vi "FestoCPX.Station.Table.Ready.vi"(7 "Log (T)":bool=TRUE, 8 "error in":errorcluster) -> (0 "error out":errorcluster, 2 "Ready state":T1)   [LabVIEW 2016]
uses:
  FestoCPX.Station.Table.ReadyState.ctl
  tools/EventLog/EventLog.EventSource.ctl
  tools/Translator/Translator.Message.ctl
  tools/EventLog/EventLog.CreateError(array).vi
  tools/Translator/Translator.Translate.Status (NoError).vi
  tools/Translator/Translator.FormatMessage.vi
  tools/Translator/Translator.Global.vi
  tools/ErrorHandling/ErrorHandling.Create.vi
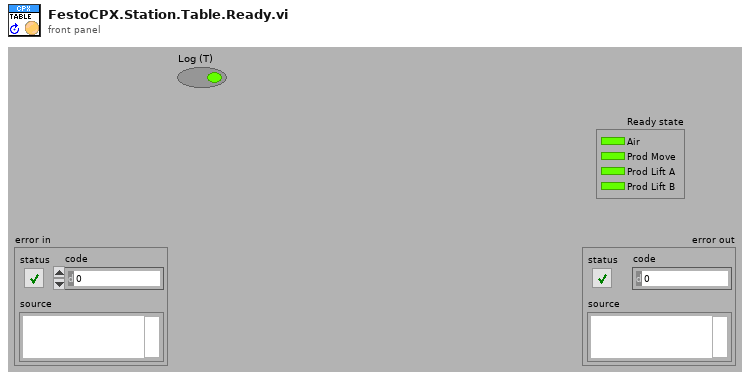
[diagram p1: front panel]
types:
  T1 = typedef "FestoCPX.Station.Table.ReadyState.ctl" = cluster{"Air":bool, "Prod Move":bool, "Prod Lift A":bool, "Prod Lift B":bool}
  T2 = typedef "EventLog.EventSource.ctl" = enum16{"All", "Gui", "Ref", "File", "Arch", "Seq", "CPX", "DB", "Laser", "Scan.P", "Scan.O"}
  T3 = typedef "Translator.Message.ctl" = enum16{"-", "Event confirmed", "Log out", "Log in", "Shutdown", "Cancel", "Start", "Begin time", "End time", "Duration", "Service Mode", "Ignore Results", "Serial Format", "On", "Off", "OK", "NOK", "NOK %s", "Home", "Work", "Close", "Open", "In progress...", "Missing", "Empty", "Hardware failure", "Initial", "Default", "Total", "Out of range", "Free disk space is below 1GB - contact technician", "Error %d >> %s", "Error %d >> %s >> %s", "Msg %d >> %s", "Laser msg %d %s", "Laser cmd error %s %d", "Laser cmd failed %s", "Laser cmd warning %s", "Laser disconnected", "Laser status %s", "Laser already started", "Laser job unkonwn %s", "Laser job missing %s", "Laser job select failure %s", "Unable to start laser printing (%s)", "Unable to stop laser printing (%s)", "Laser marking aborted", "Laser marking timeout", "Unable to reset Laser Interlock (%s)", "Unable to trigger Laser. Laser not ready (%s)", "Laser job '%s' coordinates not configured", "Starting %s", "Quitting %s", "Configured", "Initializing", "Quitting", "Loading", "Loaded %d results", "Loaded %d events", "Running", "Stopped", "Summary", "Laser", "Do you want to continue?", "Do you want to delete the configuration?", "The configuration is being used by an order. Unable to delete!", "Press confirm button", "Station is not based. Do you want to exit?", "Station requires changeover. Do you want to run the test?", "Test options are not set as default. Do you want to continue?", "Formatting of WabcoNo is disabled. Do you want to continue?", "Product not detected. Do you want to continue?", "Product scan failed. Do you want to continue?", "Calibration", "Log out?", "System", "All", "IDLE", "Translating...%s", "Not found", "Alarm %s", "Run", "Skip", "Abort", "Repeat", "Please wait...", "Database disconnected", "Database disconnected - changeover disabled!", "Login to database successful", "Login to database failed: %d; %s", "Unable to check the product status of reference %d - database disconnected", "Unable to set the product status of reference %d - database disconnected", "Variant file backup %s", "Read variant (%s)", "Result", "Station armed!", "Station requires changeover!", "Select reference number...", "EMERGENCY BUTTON - press Control button", "EMERGENCY DOOR - press Control button", "Resetting Emergency...", "Unable to reset safety circuit - Emergency Button pressed", "Unable to reset safety circuit - Emergency Side Door open", "Station not based", "Station based", "Station not empty", "Station basing...", "No order", "Press Start to begin new order", "Scanning new order", "Order NOK. Correct or scan again", "Order OK. Press Accept", "Order ready", "Revolver incorrect", "Fork incorrect", "Revolver missing", "Revolver empty", "Container missing", "Offline results", "Offline statistics", "Updating statistics %.1f %%", "DMC Configurator", "Door open", "Close the front door", "Press start button", "Done. Open the front door", "Running...", "Running...%.1f %%", "Pause %s", "Pause %s. NOK container missing", "Pause %s. OK container missing", "Pause %s. Revolver empty", "Pause %s. Revolver missing", "Pause %s. Revolver incorrect", "Pause %s. Fork missing", "Pause %s. Fork incorrect", "Pause %s. Too many failures", "Pause %s. Unloading failure", "Pause %s. One slot is not working", "Pause %s. Part order is done. Empty OK container", "Pause %s. Unable to move product to slot", "Pause %s. Unable to move back product pusher", "Pause %s. Unable to lift product", "Pause %s. Unable to move back product lifter", "Pause %s. Unable to move product arm to Work", "Pause %s. Unable to move product arm to NOK", "Pause %s. Unable to move product arm to OK", "Pause %s. Unable to unsuck the NOK product", "Pause %s. Unable to drop the NOK product", "Pause %s. Product OK missing", "Pause %s. Unable to unsuck the OK product", "Pause %s. Unable to drop the OK product", "Stopping...", "File '%s' is missing", "File '%s' is broken", "File '%s' is running", "Log file started (%s)", "Log file ended (%s)", "Log file stopped (%s)", "Log file ignored (%s)", "Log file exported (%s)", "Log file export failed (%s)", "Wrong serial number in log file", "Wrong reference number in log file", "Test steps are missing", "%s = %.3f", "Process param '%s' not found in DB", "Process param '%s' wrong order", "Process param '%s' value %.3f out of limits (%.3f; %.3f)", "Step%d param '%s' not found in DB", "Step%d param '%s' wrong order", "Step%d param '%s' value %.3f out of limits (%.3f; %.3f)", "Step%d EV '%s' not found in DB", "Step%d EV '%s' wrong order", "\"%s\" not found in DB", "\"%s\" wrong order", "\"%s\" value %.3f out of limits (%.3f; %.3f)", "\"%s\" not found in software", "Process init (%s)", "Process started", "Process restarted", "Process run", "Process done", "Process done - remove OK container", "Process aborted", "Process aborted at work", "Process aborted at home", "Process error", "Process error at home", "Process error at work", "Process close", "Process pause", "Process continue", "Process door open", "Process door close", "Process pause at slot %s due to %s", "Select plate from the order to process", "Do you want to start the process?", "Do you want to continue the process?", "There is unfinished order. Do you want to put the new order?", "Product %s %d OK", "Product %s %d NOK", "Unable to unload the slot %s. Product missing in the slot", "Unable to unload the slot %s. Product already in the arm", "Unable to accept the product as OK. Product missing in slot %s", "Unable to accept the product as OK. Product could not drop into the container at slot %s", "Unable to accept the product as NOK. Product could not drop into the container at slot %s", "Scan failed. Error %s", "Scan failed. Scanner disconnected", "Scan failed. Wrong Wabco number %d, limit (%d,%d)", "Scan failed. Wrong serial number %d, limit (%d,%d)", "Scan failed. Wrong date %d, limit (%d,%d)", "Scan failed. Wrong product wabco number %d (expected %d)", "Scan failed. Wrong product serial number %d (expected > 0)", "Scan OK %s", "Scan failed. Unable to determine table position (%s)", "Scan failed. Timeout", "Tune failed. Scanner disconnected", "Tune failed. Timeout", "%s = %d", "%s = %d->%d", "Unable to set %s = %.2f - Air Pressure Inside off", "Unable to set digital output '%s' = %d", "Unable to activate air pressure inside - timeout", "Unable to activate air pressure inside - aborted", "Unable to switch on Air Main Valve - Air Pressure Inlet off", "Unable to switch on Air Main Valve - Door open", "Unable to switch off Air Main Valve - timeout", "Unable to switch off Air Main Valve - aborted", "Unable to rotate Table - timeout", "Unable to rotate Table - aborted", "Unable to rotate Table - Product Move not in Home position", "Unable to rotate Table - Air Pressure Inside off", "Unable to rotate Table - Product Lift A not in Home position", "Unable to rotate Table - Product Lift B not in Home position", "Unable to rotate Table - unlock before movement timeout", "Unable to rotate Table - lock after movement timeout", "Unable to move Table Lock to %s position - timeout", "Unable to move Table Lock to %s position - aborted", "Unable to move Table Lock to %s position - Air Pressure Inside off", "Unable to move Table Lock to %s position - Table not in position", "Unable to move Product Lift A to %s position - timeout", "Unable to move Product Lift B to %s position - timeout", "Unable to move Product Lift A to %s position - aborted", "Unable to move Product Lift B to %s position - aborted", "Unable to move Product Lift A to %s position - Air Pressure Inside off", "Unable to move Product Lift B to %s position - Air Pressure Inside off", "Unable to move Product Lift A to %s position - Table not locked", "Unable to move Product Lift B to %s position - Table not locked", "Unable to move Product Lift A to %s position - Product Arm not in Work position", "Unable to move Product Lift B to %s position - Product Arm not in Work position", "Unable to set Product Suction Gripper %s to %s - timeout", "Unable to set Product Suction Gripper %s to %s - aborted", "Unable to set Product Suction Gripper %s to %s - Air Pressure Inside off", "Unable to set Product Suction Gripper %s to %s - Table slot unkown", "Unable to move Product Arm to %s position - timeout", "Unable to move Product Arm to %s position - aborted", "Unable to move Product Arm to %s position - Air Pressure Inside off", "Unable to move Product Arm to %s position - Product Lift A not in Home position", "Unable to move Product Arm to %s position - Product Lift B not in Home position", "Unable to move Product to %s position - timeout", "Unable to move Product to %s position - aborted", "Unable to move Product to %s position - Air Pressure Inside off", "Unable to move Product to %s position - Table not in position"}
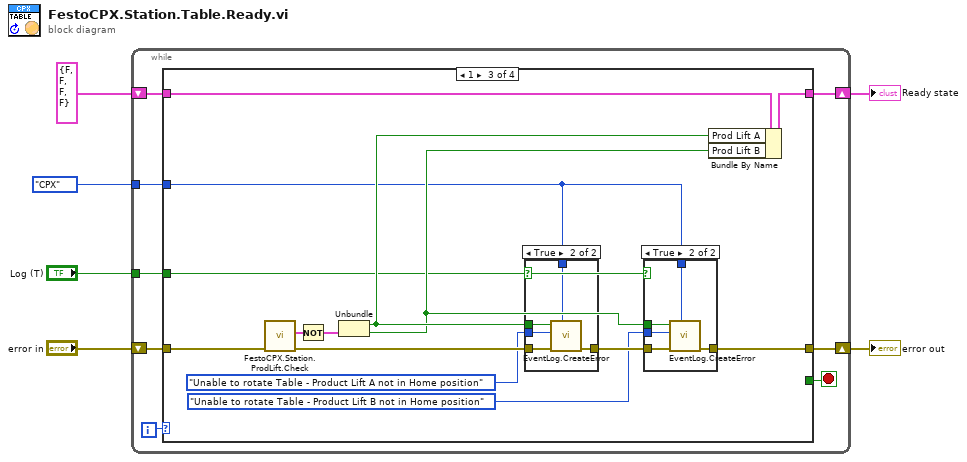
[diagram p0: block diagram]
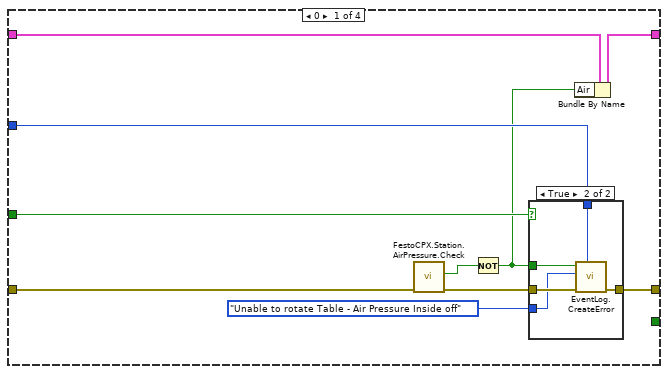
[diagram p2: hidden frame]
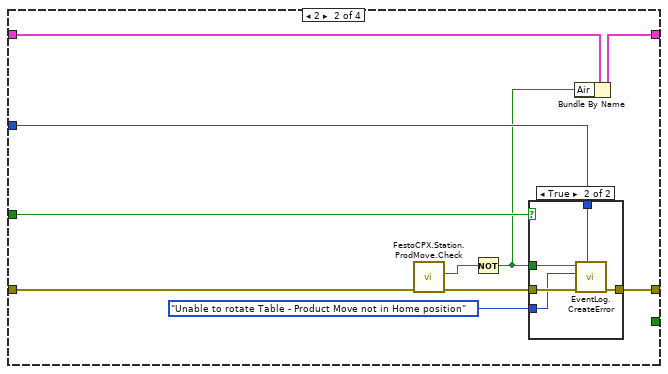
[diagram p4: hidden frame]
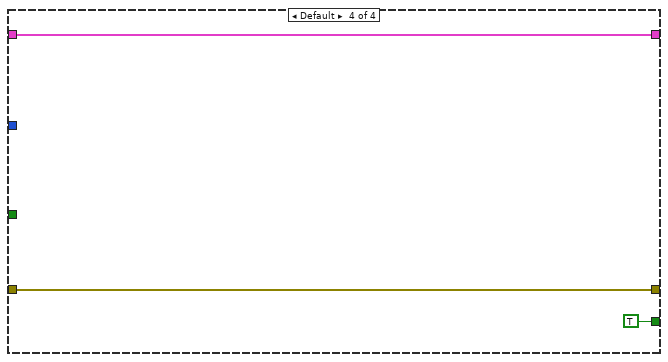
[diagram p8: hidden frame]
diagram:
  n1 = while {
    tunnel: "Log (T)" -> [w13]
    tunnel: EventLog.EventSource."CPX" ("Source") -> [w12]
    shift-right: [w7] -> w3
    shift-left: "error in" -> [w14]
    shift-right: [w8] -> w1
    shift-left: T1 {"Air"=FALSE, "Prod Move"=FALSE, "Prod Lift A"=FALSE, "Prod Lift B"=FALSE} ("Ready state") -> [w9]
    i -> [w11]
    stop <- w10 stop-if-true
    n2 = case shown="1" w11 {
      tunnel: w14 -> [w17 w33 w57 w74]
      tunnel: [w19 w35 w59 w73] -> w8
      tunnel: w13 -> [w18 w34 w52 _]
      tunnel: w12 -> [w21 w37 w50 _]
      tunnel: [_ _ _ TRUE] -> w10
      tunnel: w9 -> [w20 w36 w60 w73]
      tunnel: [w22 w38 w49 w74] -> w7
      frame 0 {
        n3 = call "FestoCPX.Station.AirPressure.Check.vi"("error in"=w17) -> ("error out"=w24:errorcluster, "Air pressure Inside"=w15:bool)  [unwired: 7 in, 2 out]
        n4 = Not(x=w15) -> (.not. x?=w16:bool)
        n5 = case shown="True" w18 {
          tunnel: w21 -> [_ w30]
          tunnel: w16 -> [_ w29]
          tunnel: w24 -> [w25 w28]
          tunnel: Translator.Message."Unable to rotate Table - Air Pressure Inside off" ("msg") -> [_ w27]
          tunnel: [w25 w26] -> w22
          frame False {
          }
          frame True {
            n6 = call-poly "EventLog.CreateError.vi"("Source (All)"=w30, "error in"=w28, "msg"=w27, "create (T)"=w29) -> ("error out"=w26:errorcluster)  [unwired: 6 in, 1 out]
          }
        }
        n7 = Bundle By Name(cluster=w20, "Air"=w16) -> (w19:T1)
      }
      frame 2 {
        n8 = call "FestoCPX.Station.ProdMove.Check.vi"("error in"=w33) -> ("error out"=w40:errorcluster, "Home"=w31:bool)  [unwired: 8 in, 1 out]
        n9 = Not(x=w31) -> (.not. x?=w32:bool)
        n10 = case shown="True" w34 {
          tunnel: w37 -> [_ w46]
          tunnel: w32 -> [_ w45]
          tunnel: w40 -> [w41 w44]
          tunnel: Translator.Message."Unable to rotate Table - Product Move not in Home position" ("msg") -> [_ w43]
          tunnel: [w41 w42] -> w38
          frame False {
          }
          frame True {
            n11 = call-poly "EventLog.CreateError.vi"("Source (All)"=w46, "error in"=w44, "msg"=w43, "create (T)"=w45) -> ("error out"=w42:errorcluster)  [unwired: 6 in, 1 out]
          }
        }
        n12 = Bundle By Name(cluster=w36, "Air"=w32) -> (w35:T1)
      }
      frame 1 {
        n13 = call "FestoCPX.Station.ProdLift.Check.vi"("error in"=w57) -> ("error out"=w58:errorcluster, "Home"=w56:cluster{"A":bool, "B":bool})  [unwired: 8 in, 1 out]
        n14 = Not(x=w56) -> (.not. x?=w54:cluster{"A":bool, "B":bool})
        n15 = Unbundle(w54) -> ("A"=w55:bool, "B"=w53:bool)
        n16 = case shown="True" w52 {
          tunnel: w50 -> [_ w72]
          tunnel: w55 -> [_ w71]
          tunnel: w58 -> [w67 w70]
          tunnel: Translator.Message."Unable to rotate Table - Product Lift A not in Home position" ("msg") -> [_ w69]
          tunnel: [w67 w68] -> w51
          frame False {
          }
          frame True {
            n17 = call-poly "EventLog.CreateError.vi"("Source (All)"=w72, "error in"=w70, "msg"=w69, "create (T)"=w71) -> ("error out"=w68:errorcluster)  [unwired: 6 in, 1 out]
          }
        }
        n18 = case shown="True" w52 {
          tunnel: w50 -> [_ w66]
          tunnel: w53 -> [_ w65]
          tunnel: w51 -> [w61 w64]
          tunnel: Translator.Message."Unable to rotate Table - Product Lift B not in Home position" ("msg") -> [_ w63]
          tunnel: [w61 w62] -> w49
          frame False {
          }
          frame True {
            n19 = call-poly "EventLog.CreateError.vi"("Source (All)"=w66, "error in"=w64, "msg"=w63, "create (T)"=w65) -> ("error out"=w62:errorcluster)  [unwired: 6 in, 1 out]
          }
        }
        n20 = Bundle By Name(cluster=w60, "Prod Lift A"=w55, "Prod Lift B"=w53) -> (w59:T1)
      }
      frame Default {
      }
    }
  }
  "error out" <- w3
  "Ready state" <- w1
